vi "ToRawCommands.vi"(1 "Macro Info 2D":T1(array[cluster])=[[{"Duration (s)"=0.01, "Instruction Description"="Initial state", "Input Bits"=[FALSE, FALSE, FALSE, FALSE, FALSE, FALSE, FALSE, FALSE, FALSE, FALSE, FALSE, FALSE, FALSE, FALSE, FALSE, FALSE], "Output Bits"=[FALSE, FALSE, FALSE, FALSE, FALSE, FALSE, FALSE, FALSE, FALSE, FALSE, FALSE, FALSE, FALSE, FALSE, FALSE, FALSE, FALSE, FALSE, FALSE, FALSE, FALSE, FALSE, FALSE, FALSE, FALSE, FALSE, FALSE, FALSE, FALSE, FALSE, FALSE, FALSE, FALSE, FALSE, FALSE, FALSE, FALSE, FALSE], "Excitations"=[0.006641157877225088, -1.3304949441192124e-05, -1.3273425937601626e-05, -6.65619425437312e-06, -6.648715135800007e-06, -6.648052120728627e-06, -6.652961565841034e-06, -0.0001659795114891018, 0.0, 0.0, 0.0, 0.0, 0.0, 0.0, 0.0, 0.0], "Steps"=1, "Changes"=[FALSE, TRUE, TRUE]}, {"Duration (s)"=0.01, "Instruction Description"="Blocking potentials", "Input Bits"=[FALSE, FALSE, FALSE, FALSE, FALSE, FALSE, FALSE, FALSE, FALSE, FALSE, FALSE, FALSE, FALSE, FALSE, FALSE, FALSE], "Output Bits"=[FALSE, FALSE, FALSE, FALSE, FALSE, FALSE, FALSE, FALSE, FALSE, FALSE, FALSE, FALSE, FALSE, FALSE, FALSE, FALSE, FALSE, FALSE, FALSE, FALSE, FALSE, FALSE, FALSE, FALSE, FALSE, FALSE, FALSE, FALSE, FALSE, FALSE, FALSE, FALSE, FALSE, FALSE, FALSE, FALSE, FALSE, FALSE], "Excitations"=[-4.658140076526369, -1.3304949441192124e-05, -1.3273425937601626e-05, -6.65619425437312e-06, -6.648715135800007e-06, -5.318448344635022, -5.322375905634393, -0.0001659795114891018, 0.0, 0.0, 0.0, 0.0, 0.0, 0.0, 0.0, 0.0], "Steps"=1, "Changes"=[FALSE, FALSE, TRUE]}, {"Duration (s)"=0.005, "Instruction Description"="Enable e- source", "Input Bits"=[FALSE, FALSE, FALSE, FALSE, FALSE, FALSE, FALSE, FALSE, FALSE, FALSE, FALSE, FALSE, FALSE, FALSE, FALSE, FALSE], "Output Bits"=[FALSE, FALSE, FALSE, FALSE, FALSE, FALSE, FALSE, FALSE, FALSE, TRUE, FALSE, FALSE, FALSE, FALSE, FALSE, FALSE, FALSE, FALSE, FALSE, FALSE, FALSE, FALSE, FALSE, FALSE, FALSE, FALSE, FALSE, FALSE, FALSE, FALSE, FALSE, FALSE, FALSE, FALSE, FALSE, FALSE, FALSE, FALSE], "Excitations"=[-4.658140076526369, -1.3304949441192124e-05, -1.3273425937601626e-05, -6.65619425437312e-06, -6.648715135800007e-06, -5.318448344635022, -5.322375905634393, -0.0001659795114891018, 0.0, 0.0, 0.0, 0.0, 0.0, 0.0, 0.0, 0.0], "Steps"=1, "Changes"=[FALSE, TRUE, FALSE]}, {"Duration (s)"=0.02, "Instruction Description"="Open US side", "Input Bits"=[FALSE, FALSE, FALSE, FALSE, FALSE, FALSE, FALSE, FALSE, FALSE, FALSE, FALSE, FALSE, FALSE, FALSE, FALSE, FALSE], "Output Bits"=[FALSE, FALSE, FALSE, FALSE, FALSE, FALSE, FALSE, FALSE, FALSE, TRUE, FALSE, FALSE, FALSE, FALSE, FALSE, FALSE, FALSE, FALSE, FALSE, FALSE, FALSE, FALSE, FALSE, FALSE, FALSE, FALSE, FALSE, FALSE, FALSE, FALSE, FALSE, FALSE, FALSE, FALSE, FALSE, FALSE, FALSE, FALSE], "Excitations"=[-1.3308933621693563e-05, -1.3304949441192124e-05, -1.3273425937601626e-05, -6.65619425437312e-06, -6.648715135800007e-06, -5.318448344635022, -5.322375905634393, -0.0001659795114891018, 0.0, 0.0, 0.0, 0.0, 0.0, 0.0, 0.0, 0.0], "Steps"=1, "Changes"=[FALSE, FALSE, TRUE]}, {"Duration (s)"=5.0, "Instruction Description"="5 s pulldown", "Input Bits"=[FALSE, FALSE, FALSE, FALSE, FALSE, FALSE, FALSE, FALSE, FALSE, FALSE, FALSE, FALSE, FALSE, FALSE, FALSE, FALSE], "Output Bits"=[FALSE, FALSE, FALSE, FALSE, FALSE, FALSE, FALSE, FALSE, FALSE, TRUE, FALSE, FALSE, FALSE, FALSE, FALSE, FALSE, FALSE, FALSE, FALSE, FALSE, FALSE, FALSE, FALSE, FALSE, FALSE, FALSE, FALSE, FALSE, FALSE, FALSE, FALSE, FALSE, FALSE, FALSE, FALSE, FALSE, FALSE, FALSE], "Excitations"=[-1.3308933621693563e-05, 5.9872139435870135, 5.309357101614712, 5.324948747304241, 5.318965459924869, -5.318448344635022, -5.322375905634393, -0.0001659795114891018, 0.0, 0.0, 0.0, 0.0, 0.0, 0.0, 0.0, 0.0], "Steps"=1000, "Changes"=[FALSE, FALSE, TRUE]}, {"Duration (s)"=0.025, "Instruction Description"="Barn door", "Input Bits"=[FALSE, FALSE, FALSE, FALSE, FALSE, FALSE, FALSE, FALSE, FALSE, FALSE, FALSE, FALSE, FALSE, FALSE, FALSE, FALSE], "Output Bits"=[FALSE, FALSE, FALSE, FALSE, FALSE, FALSE, FALSE, FALSE, FALSE, TRUE, FALSE, FALSE, FALSE, FALSE, FALSE, FALSE, FALSE, FALSE, FALSE, FALSE, FALSE, FALSE, FALSE, FALSE, FALSE, FALSE, FALSE, FALSE, FALSE, FALSE, FALSE, FALSE, FALSE, FALSE, FALSE, FALSE, FALSE, FALSE], "Excitations"=[-5.3235867576110465, 5.9872139435870135, 5.309357101614712, 5.324948747304241, 5.318965459924869, -5.318448344635022, -5.322375905634393, -0.0001659795114891018, 0.0, 0.0, 0.0, 0.0, 0.0, 0.0, 0.0, 0.0], "Steps"=1, "Changes"=[FALSE, FALSE, TRUE]}, {"Duration (s)"=0.5, "Instruction Description"="Disable e- source and move over", "Input Bits"=[FALSE, FALSE, FALSE, FALSE, FALSE, FALSE, FALSE, FALSE, FALSE, FALSE, FALSE, FALSE, FALSE, FALSE, FALSE, FALSE], "Output Bits"=[FALSE, FALSE, FALSE, FALSE, FALSE, FALSE, FALSE, FALSE, FALSE, FALSE, FALSE, FALSE, FALSE, FALSE, FALSE, FALSE, FALSE, FALSE, FALSE, FALSE, FALSE, FALSE, FALSE, FALSE, FALSE, FALSE, FALSE, FALSE, FALSE, FALSE, FALSE, FALSE, FALSE, FALSE, FALSE, FALSE, FALSE, FALSE], "Excitations"=[-6.654480119780403, 6.65246141564662, 6.636699695374874, 6.656187598178865, -6.648721784515143, -6.648058768780747, -6.6529682188026, -0.0001659795114891018, 0.0, 0.0, 0.0, 0.0, 0.0, 0.0, 0.0, 0.0], "Steps"=100, "Changes"=[FALSE, TRUE, TRUE]}], [{"Duration (s)"=1.0, "Instruction Description"="Disable Tanaka", "Input Bits"=[FALSE, FALSE, FALSE, FALSE, FALSE, FALSE, FALSE, FALSE, FALSE, FALSE, FALSE, FALSE, FALSE, FALSE, FALSE, FALSE], "Output Bits"=[FALSE, FALSE, FALSE, FALSE, FALSE, FALSE, FALSE, FALSE, FALSE, FALSE, FALSE, FALSE, FALSE, FALSE, FALSE, FALSE, FALSE, FALSE, FALSE, FALSE, FALSE, FALSE, FALSE, FALSE, FALSE, FALSE, FALSE, FALSE, FALSE, FALSE, FALSE, FALSE, FALSE, FALSE, FALSE, FALSE, FALSE, FALSE], "Excitations"=[-6.654480119780403, 6.65246141564662, 6.636699695374874, 6.656187598178865, -6.648721784515143, -6.648058768780747, -6.6529682188026, -0.0001659795114891018, 0.0, 0.0, 0.0, 0.0, 0.0, 0.0, 0.0, 0.0], "Steps"=1, "Changes"=[FALSE, TRUE, TRUE]}, {"Duration (s)"=0.0, "Instruction Description"="", "Input Bits"=[], "Output Bits"=[], "Excitations"=[], "Steps"=0, "Changes"=[]}, {"Duration (s)"=0.0, "Instruction Description"="", "Input Bits"=[], "Output Bits"=[], "Excitations"=[], "Steps"=0, "Changes"=[]}, {"Duration (s)"=0.0, "Instruction Description"="", "Input Bits"=[], "Output Bits"=[], "Excitations"=[], "Steps"=0, "Changes"=[]}, {"Duration (s)"=0.0, "Instruction Description"="", "Input Bits"=[], "Output Bits"=[], "Excitations"=[], "Steps"=0, "Changes"=[]}, {"Duration (s)"=0.0, "Instruction Description"="", "Input Bits"=[], "Output Bits"=[], "Excitations"=[], "Steps"=0, "Changes"=[]}, {"Duration (s)"=0.0, "Instruction Description"="", "Input Bits"=[], "Output Bits"=[], "Excitations"=[], "Steps"=0, "Changes"=[]}], [{"Duration (s)"=0.001, "Instruction Description"="Initial state", "Input Bits"=[FALSE, FALSE, FALSE, FALSE, FALSE, FALSE, FALSE, FALSE, FALSE, FALSE, FALSE, FALSE, FALSE, FALSE, FALSE, FALSE], "Output Bits"=[FALSE, FALSE, FALSE, FALSE, FALSE, FALSE, FALSE, FALSE, FALSE, FALSE, FALSE, FALSE, FALSE, FALSE, FALSE, FALSE, FALSE, FALSE, FALSE, FALSE, FALSE, FALSE, FALSE, FALSE, FALSE, FALSE, FALSE, FALSE, FALSE, FALSE, FALSE, FALSE, FALSE, FALSE, FALSE, FALSE, FALSE, FALSE], "Excitations"=[-6.654480119780403, 6.65246141564662, 6.636699695374874, 6.656187598178865, -6.648721784515143, -6.648058768780747, -6.6529682188026, -0.0001659795114891018, 0.0, 0.0, 0.0, 0.0, 0.0, 0.0, 0.0, 0.0], "Steps"=1, "Changes"=[FALSE, TRUE, TRUE]}, {"Duration (s)"=0.1, "Instruction Description"="Raise well", "Input Bits"=[FALSE, FALSE, FALSE, FALSE, FALSE, FALSE, FALSE, FALSE, FALSE, FALSE, FALSE, FALSE, FALSE, FALSE, FALSE, FALSE], "Output Bits"=[FALSE, FALSE, FALSE, FALSE, FALSE, FALSE, FALSE, FALSE, FALSE, FALSE, FALSE, FALSE, FALSE, FALSE, FALSE, FALSE, FALSE, FALSE, FALSE, FALSE, FALSE, FALSE, FALSE, FALSE, FALSE, FALSE, FALSE, FALSE, FALSE, FALSE, FALSE, FALSE, FALSE, FALSE, FALSE, FALSE, FALSE, FALSE], "Excitations"=[-7.985373481949759, -5.854191059073976, -6.63672624222675, -6.6562009105673745, -7.978464811675144, -7.977669192926473, -7.983560531970807, -0.0001659795114891018, 0.0, 0.0, 0.0, 0.0, 0.0, 0.0, 0.0, 0.0], "Steps"=1000, "Changes"=[FALSE, FALSE, TRUE]}, {"Duration (s)"=0.01, "Instruction Description"="Wait 10 ms", "Input Bits"=[FALSE, FALSE, FALSE, FALSE, FALSE, FALSE, FALSE, FALSE, FALSE, FALSE, FALSE, FALSE, FALSE, FALSE, FALSE, FALSE], "Output Bits"=[FALSE, FALSE, FALSE, FALSE, FALSE, FALSE, FALSE, FALSE, FALSE, FALSE, FALSE, FALSE, FALSE, FALSE, FALSE, FALSE, FALSE, FALSE, FALSE, FALSE, FALSE, FALSE, FALSE, FALSE, FALSE, FALSE, FALSE, FALSE, FALSE, FALSE, FALSE, FALSE, FALSE, FALSE, FALSE, FALSE, FALSE, FALSE], "Excitations"=[-7.985373481949759, -5.854191059073976, -6.63672624222675, -6.6562009105673745, -7.978464811675144, -7.977669192926473, -7.983560531970807, -0.0001659795114891018, 0.0, 0.0, 0.0, 0.0, 0.0, 0.0, 0.0, 0.0], "Steps"=1, "Changes"=[FALSE, FALSE, FALSE]}, {"Duration (s)"=0.0, "Instruction Description"="", "Input Bits"=[], "Output Bits"=[], "Excitations"=[], "Steps"=0, "Changes"=[]}, {"Duration (s)"=0.0, "Instruction Description"="", "Input Bits"=[], "Output Bits"=[], "Excitations"=[], "Steps"=0, "Changes"=[]}, {"Duration (s)"=0.0, "Instruction Description"="", "Input Bits"=[], "Output Bits"=[], "Excitations"=[], "Steps"=0, "Changes"=[]}, {"Duration (s)"=0.0, "Instruction Description"="", "Input Bits"=[], "Output Bits"=[], "Excitations"=[], "Steps"=0, "Changes"=[]}], [{"Duration (s)"=0.001, "Instruction Description"="Initial state", "Input Bits"=[FALSE, FALSE, FALSE, FALSE, FALSE, FALSE, FALSE, FALSE, FALSE, FALSE, FALSE, FALSE, FALSE, FALSE, FALSE, FALSE], "Output Bits"=[FALSE, FALSE, FALSE, FALSE, FALSE, FALSE, FALSE, FALSE, FALSE, FALSE, FALSE, FALSE, FALSE, FALSE, FALSE, FALSE, FALSE, FALSE, FALSE, FALSE, FALSE, FALSE, FALSE, FALSE, FALSE, FALSE, FALSE, FALSE, FALSE, FALSE, FALSE, FALSE, FALSE, FALSE, FALSE, FALSE, FALSE, FALSE], "Excitations"=[-7.985373481949759, -5.854191059073976, -6.63672624222675, -6.6562009105673745, -7.978464811675144, -7.977669192926473, -7.983560531970807, -0.0001659795114891018, 0.0, 0.0, 0.0, 0.0, 0.0, 0.0, 0.0, 0.0], "Steps"=1, "Changes"=[FALSE, TRUE, TRUE]}, {"Duration (s)"=0.05, "Instruction Description"="DAQ trig and raise a disconnected DAC line", "Input Bits"=[FALSE, FALSE, FALSE, FALSE, FALSE, FALSE, FALSE, FALSE, FALSE, FALSE, FALSE, FALSE, FALSE, FALSE, FALSE, FALSE], "Output Bits"=[TRUE, FALSE, FALSE, FALSE, FALSE, FALSE, FALSE, FALSE, FALSE, FALSE, FALSE, FALSE, FALSE, FALSE, FALSE, FALSE, FALSE, FALSE, FALSE, FALSE, FALSE, FALSE, FALSE, FALSE, FALSE, FALSE, FALSE, FALSE, FALSE, FALSE, FALSE, FALSE, FALSE, FALSE, FALSE, FALSE, FALSE, FALSE], "Excitations"=[-7.852284145732824, -6.6524880255455034, -6.63672624222675, -6.6562009105673745, -7.978464811675144, -7.977669192926473, -7.983560531970807, -0.0001659795114891018, 0.0, 0.0, 0.0, 0.0, 0.0, 0.0, 0.0, 0.6666666666666666], "Steps"=500, "Changes"=[FALSE, TRUE, TRUE]}, {"Duration (s)"=0.0, "Instruction Description"="", "Input Bits"=[], "Output Bits"=[], "Excitations"=[], "Steps"=0, "Changes"=[]}, {"Duration (s)"=0.0, "Instruction Description"="", "Input Bits"=[], "Output Bits"=[], "Excitations"=[], "Steps"=0, "Changes"=[]}, {"Duration (s)"=0.0, "Instruction Description"="", "Input Bits"=[], "Output Bits"=[], "Excitations"=[], "Steps"=0, "Changes"=[]}, {"Duration (s)"=0.0, "Instruction Description"="", "Input Bits"=[], "Output Bits"=[], "Excitations"=[], "Steps"=0, "Changes"=[]}, {"Duration (s)"=0.0, "Instruction Description"="", "Input Bits"=[], "Output Bits"=[], "Excitations"=[], "Steps"=0, "Changes"=[]}]], 2 "# AO cards":u8=2) -> (0 "RAW cluster":cluster{i16[][]}[][](array[cluster])=[[{[[22, 0, 0, 0, 0, 0, 0, -1, 22, 0, 0, 0, 0, 0, 0, -1], [0, 0, 0, 0, 0, 0, 0, 0, 0, 0, 0, 0, 0, 0, 0, 0]]}, {[[-15264, 0, 0, 0, 0, -17427, -17440, -1, -15264, 0, 0, 0, 0, -17427, -17440, -1], [0, 0, 0, 0, 0, 0, 0, 0, 0, 0, 0, 0, 0, 0, 0, 0]]}, {[[-15264, 0, 0, 0, 0, -17427, -17440, -1, -15264, 0, 0, 0, 0, -17427, -17440, -1], [0, 0, 0, 0, 0, 0, 0, 0, 0, 0, 0, 0, 0, 0, 0, 0]]}, {[[0, 0, 0, 0, 0, -17427, -17440, -1, 0, 0, 0, 0, 0, -17427, -17440, -1], [0, 0, 0, 0, 0, 0, 0, 0, 0, 0, 0, 0, 0, 0, 0, 0]]}, {array2x8000[16000 elements]}, {[[-17444, 19619, 17398, 17449, 17429, -17427, -17440, -1, -17444, 19619, 17398, 17449, 17429, -17427, -17440, -1], [0, 0, 0, 0, 0, 0, 0, 0, 0, 0, 0, 0, 0, 0, 0, 0]]}, {array2x800[1600 elements]}], [{[[-21805, 21799, 21747, 21811, -21787, -21784, -21800, -1, -21805, 21799, 21747, 21811, -21787, -21784, -21800, -1], [0, 0, 0, 0, 0, 0, 0, 0, 0, 0, 0, 0, 0, 0, 0, 0]]}, {[]}, {[]}, {[]}, {[]}, {[]}, {[]}], [{[[-21805, 21799, 21747, 21811, -21787, -21784, -21800, -1, -21805, 21799, 21747, 21811, -21787, -21784, -21800, -1], [0, 0, 0, 0, 0, 0, 0, 0, 0, 0, 0, 0, 0, 0, 0, 0]]}, {array2x8000[16000 elements]}, {[[-26166, -19183, -21747, -21811, -26144, -26141, -26161, -1, -26166, -19183, -21747, -21811, -26144, -26141, -26161, -1], [0, 0, 0, 0, 0, 0, 0, 0, 0, 0, 0, 0, 0, 0, 0, 0]]}, {[]}, {[]}, {[]}, {[]}], [{[[-26166, -19183, -21747, -21811, -26144, -26141, -26161, -1, -26166, -19183, -21747, -21811, -26144, -26141, -26161, -1], [0, 0, 0, 0, 0, 0, 0, 0, 0, 0, 0, 0, 0, 0, 0, 0]]}, {array2x4000[8000 elements]}, {[]}, {[]}, {[]}, {[]}, {[]}]])   [LabVIEW 2018]
uses:
  <vilib>/Analysis/1siggen.llb/Ramp Pattern by Samples.vi
  <vilib>/Analysis/NI_AALBase.lvlib
panel:
  out "Last Excitations":dbl[](array[numeric])=[-7.852284145732824, -6.6524880255455034, -6.63672624222675, -6.6562009105673745, -7.978464811675144, -7.977669192926473, -7.983560531970807, -0.0001659795114891018, 0.0, 0.0, 0.0, 0.0, 0.0, 0.0, 0.0, 0.6666666666666666]
  out "Instruction":i32=6
  out "Action":i32=3
  # "RAW cmds: array of voltage ints, for each card, for each Instruction, for each Action\n\nIn other words\nRAW cmds:\n  Actions\n  |- Instructions\n      |-  AO cards\n           |-  integer arrays"
  # "Action"
  # "Instruction"
  # "AO card"
  # "RAWindex"
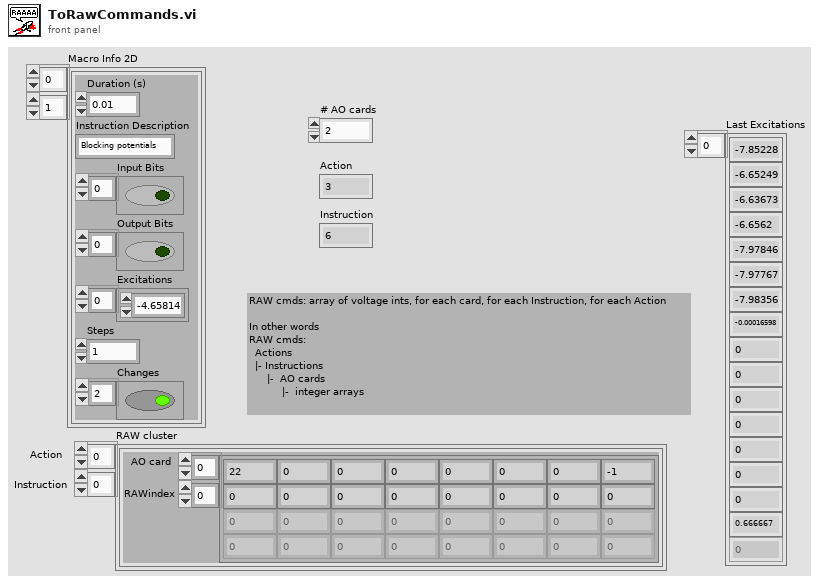
[diagram p1: front panel]
types:
  T1 = cluster{"Duration (s)":dbl, "Instruction Description":string, "Input Bits":bool[], "Output Bits":bool[], "Excitations":dbl[], "Steps":i32, "Changes":bool[]}[][]
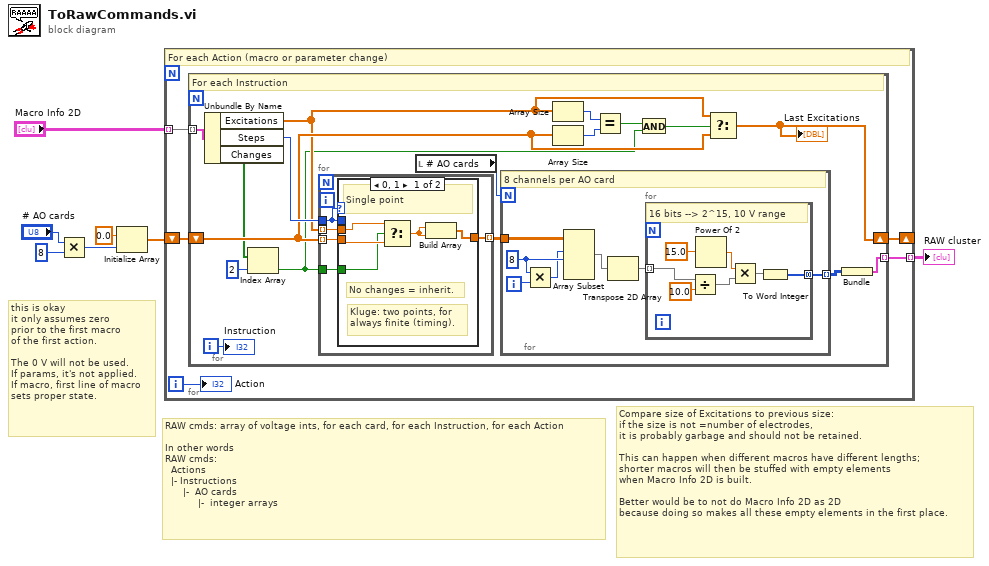
[diagram p0: block diagram]
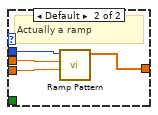
[diagram p2: hidden frame]
diagram:
  # "Compare size of Excitations to previous size:\nif the size is not =number of electrodes, \nit is probably garbage and should not be retained.\n\nThis can happen when different macros have different lengths;\nshorter macros will then be stuffed with empty elements\nwhen Macro Info 2D is built.\n\nBetter would be to not do Macro Info 2D as 2D\nbecause doing so makes all these empty elements in the first place."
  # "this is okay\nit only assumes zero\nprior to the first macro\nof the first action.\n\nThe 0 V will not be used.\nIf params, it's not applied.\nIf macro, first line of macro\nsets proper state."
  # "RAW cmds: array of voltage ints, for each card, for each Instruction, for each Action\n\nIn other words\nRAW cmds:\n  Actions\n  |- Instructions\n      |-  AO cards\n           |-  integer arrays"
  n1 = Multiply(x="# AO cards", y=8) -> (x*y=w2:i32)
  n2 = Initialize Array(0.0 ("element"), w2) -> (w6:dbl[])
  n3 = for {
    tunnel: "Macro Info 2D" -> [w10] mode=indexing
    shift-right: [w11] -> _
    shift-left: w6 -> [w12]
    tunnel: [w9] -> w1 mode=indexing
    i -> [w8]
    # "For each Action (macro or parameter change)"
    n4 = for {
      tunnel: w10 -> [w29] mode=indexing
      shift-right: [w20] -> w11
      shift-left: w12 -> [w19]
      tunnel: [w25] -> w9 mode=indexing
      i -> [w23]
      # "For each Instruction"
      n5 = Unbundle By Name(w29) -> ("Excitations"=w18:dbl[], "Steps"=w28:i32, "Changes"=w17:bool[])
      n6 = Index Array(array=w17, index=2) -> (element=w15:bool)
      n7 = for {
        tunnel: w19 -> [w48] mode=indexing
        tunnel: w18 -> [w47] mode=indexing
        tunnel: w28 -> [w45]
        tunnel: [w46] -> w27 mode=indexing
        tunnel: w15 -> [w44]
        n8 = case shown="0, 1" w45 {
          tunnel: w48 -> [w50 w57]
          tunnel: w47 -> [w51 w56]
          tunnel: w45 -> [_ w55]
          tunnel: [w53 w54] -> w46
          tunnel: w44 -> [w49 _]
          frame 0, 1 {
            # "Kluge: two points, for \nalways finite (timing)."
            # "No changes = inherit."
            # "Single point"
            n9 = Select(t=w51, s=w49, f=w50) -> (s? t:f=w52:dbl)
            n10 = Build Array(w52, w52) -> (w53:dbl[])
          }
          frame Default {
            # "Actually a ramp"
            n11 = call-poly <vilib>:"Ramp Pattern.vi"("start"=w57, "end"=w56, "samples"=w55) -> ("Ramp Pattern"=w54:dbl[])  [unwired: 7 in, 1 out]
          }
        }
      }
      n12 = local read "# AO cards"() -> (w26:u8)
      n13 = for {
        N: w26 -> [_]
        tunnel: w27 -> [w36]
        tunnel: [w31] -> w24 mode=indexing
        i -> [w35]
        w34 = 8 ("length")
        # "8 channels per AO card"
        n14 = Multiply(x=w34, y=w35) -> (x*y=w33:i32)
        n15 = Array Subset(array=w36, index (row)=w33, length (row)=w34) -> (w30:dbl[][])  [unwired: 2 in]
        n16 = Transpose 2D Array(2D array=w30) -> (transposed array=w32:dbl[][])
        n17 = for {
          tunnel: w32 -> [w38] mode=indexing
          tunnel: [w37] -> w31 mode=concatenating
          # "16 bits --> 2^15, 10 V range"
          n18 = Divide(x=w38, y=10.0) -> (x/y=w43:dbl[])
          n19 = Power Of 2(x=15.0) -> (2^x=w42:dbl)
          n20 = Multiply(x=w42, y=w43) -> (x*y=w41:dbl[])
          n21 = To Word Integer(number=w41) -> (16bit integer=w37:i16[])
        }
      }
      n22 = Array Size(array=w18) -> (size(s)=w22:i32)
      n23 = Array Size(array=w19) -> (size(s)=w21:i32)
      n24 = Equal?(x=w22, y=w21) -> (x = y?=w16:bool)
      n25 = And(x=w16, y=w15) -> (x .and. y?=w14:bool)
      n26 = Select(t=w18, s=w14, f=w19) -> (s? t:f=w20:dbl[])
      "Last Excitations" <- w20
      n27 = Bundle(w24) -> (w25:cluster{i16[][]})  [unwired: 1 in]
      "Instruction" <- w23
    }
    "Action" <- w8
  }
  "RAW cluster" <- w1
